vi "TSM Scope Close Sessions.vi"(0 "TSM context":T1) -> (15 "error out":errorcluster)   [LabVIEW 2020]
doc: "Use this VI to reset and close all sessions for all NI-SCOPE instruments in the Semiconductor Module Context."
uses:
  <vilib>/NI_TestStand_SemiconductorModule/NI_TestStand_Semiconductor_Module.lvlibp/PinMap/General/SemiconductorModuleContext.ctl
  <vilib>/NI_TestStand_SemiconductorModule/NI_TestStand_Semiconductor_Module.lvlibp
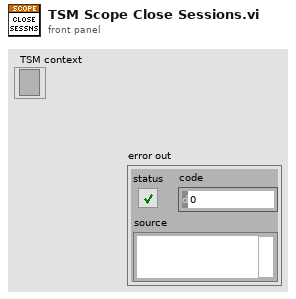
[diagram p1: front panel]
types:
  T1 = typedef "NI_TestStand_Semiconductor_Module.lvlibp/SemiconductorModuleContext.ctl" = refnum<k7>
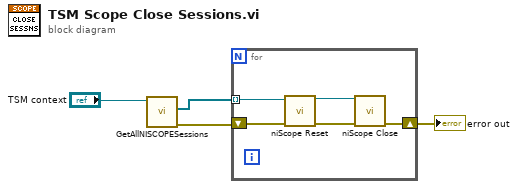
[diagram p0: block diagram]
diagram:
  n1 = call <vilib>:"GetAllNISCOPESessions.vi"("Semiconductor Module Context"="TSM context") -> ("error out"=w3:errorcluster, "Instrument Sessions"=w2:refnum<k15>[])  [unwired: 8 in, 1 out]
  n2 = for {
    tunnel: w2 -> [w6] mode=indexing
    shift-right: [w8] -> w4
    shift-left: w3 -> [w9]
    n3 = call <instrlib>:"niScope Reset.vi"("instrument handle"=w6, "error in"=w9) -> ("instrument handle out"=w5:refnum<k15>, "error out"=w7:errorcluster)  [unwired: 12 in]
    n4 = call <instrlib>:"niScope Close.vi"("instrument handle"=w5, "error in"=w7) -> ("error out"=w8:errorcluster)  [unwired: 13 in]
  }
  "error out" <- w4
